vi "IncludeFile.vi"(8 "error in (no error)":errorcluster, 10 "Path":path, 11 "Whitelist in":refnum<class "Whitelist.lvclass">) -> (0 "error out":errorcluster, 3 "Whitelist out":refnum<class "Whitelist.lvclass">)   [LabVIEW 2019, in "Whitelist.lvclass"]
doc: "Includes a single file in the whitelist."
uses:
  Whitelist.lvclass
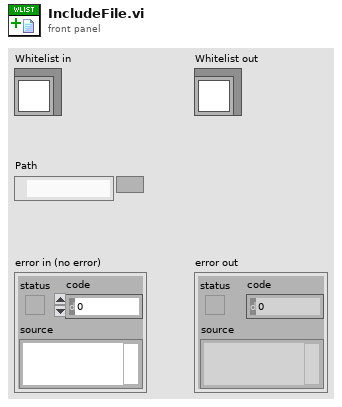
[diagram p1: front panel]
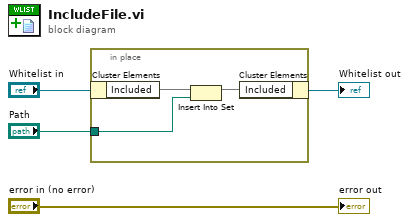
[diagram p0: block diagram]
diagram:
  n1 = in-place {
    in-place-border: "Path" -> [w6]
    n2 = in-place-cluster #1("Whitelist in") -> ("Included"=w7:set{path})
    n3 = Insert Into Set(10:w6, 11:w7) -> (3:w5:set{path})  [unwired: 1 out]
    n4 = in-place-cluster #1("Included"=w5) -> (→"Whitelist out":refnum<class "Whitelist.lvclass">)
  }
  "error out" <- "error in (no error)"
